vi "BL Calc Fourier.vi"(4 "EMF":dbl[](array[numeric]), 6 "cap probe":dbl[](array[numeric]), 10 "Period (us)":i64, 11 "FREQU":dbl) -> (2 "velocity":dbl, 3 "EMF":dbl)   [LabVIEW 2018]
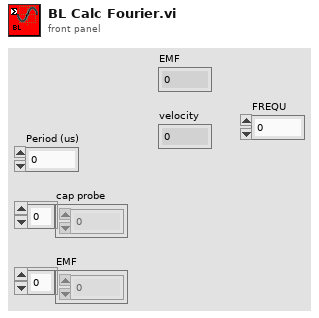
[diagram p1: front panel]
types:
  T1 = typedef "Fourier Outputs.ctl" = cluster{"Time period":dbl, "computed \namplitude":dbl, "number of cycles":dbl}
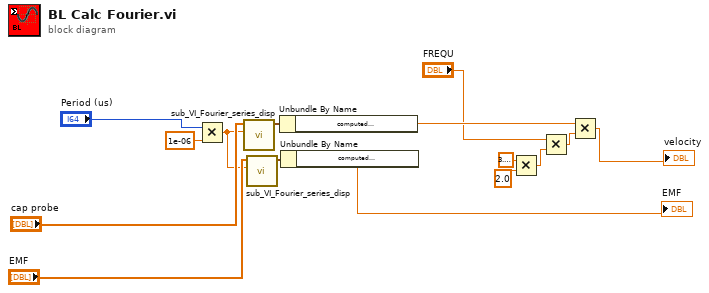
[diagram p0: block diagram]
diagram:
  n1 = Multiply(x="Period (us)", y=1e-06) -> (x*y=w8:dbl)
  n2 = call "sub_VI_Fourier_series_disp.vi"("del t"=w8, "x,i"="cap probe") -> ("outputs"=w12:T1)  [unwired: 8 in, 1 out]
  n3 = call "sub_VI_Fourier_series_disp.vi"("del t"=w8, "x,i"="EMF") -> ("outputs"=w13:T1)  [unwired: 8 in, 1 out]
  n4 = Unbundle By Name(w12) -> ("computed \namplitude"=w14:dbl)
  n5 = Unbundle By Name(w13) -> ("computed \namplitude"=→"EMF":dbl)
  n6 = Multiply(x=3.141592653589793, y=2.0) -> (x*y=w4:dbl)
  n7 = Multiply(x="FREQU", y=w4) -> (x*y=w7:dbl)
  n8 = Multiply(x=w14, y=w7) -> (x*y=→"velocity":dbl)
